vi "niDTS WLAN UTIL chains to chains array.vi"(10 "Chains":T1) -> (2 "Chains Array":bool[](array[boolean])=[TRUE, FALSE, FALSE, FALSE])   [LabVIEW 2014, in "niDTS WLAN.lvlib"]
uses:
  niDTS WLAN.lvlib
  Includes/niDTS WLAN INC Chains.ctl
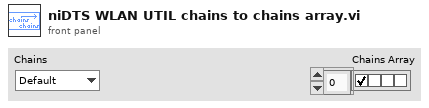
[diagram p1: front panel]
types:
  T1 = typedef "niDTS WLAN.lvlib/niDTS WLAN INC Chains.ctl" = enum16{"Default", "Chain 0", "Chain 1", "Chain 2", "Chain 3", "Chain 0 and 1", "Chain 2 and 3", "Chain 1,2 and 3", "Chains 1 - 4"}
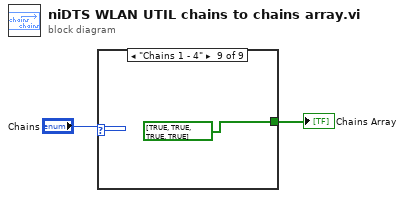
[diagram p0: block diagram]
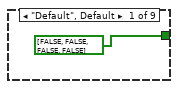
[diagram p2: hidden frame]
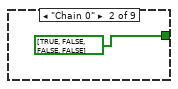
[diagram p3: hidden frame]
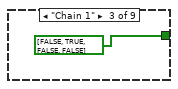
[diagram p4: hidden frame]
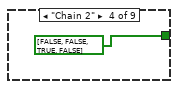
[diagram p5: hidden frame]
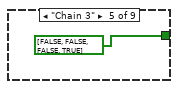
[diagram p6: hidden frame]
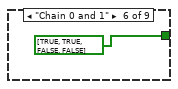
[diagram p7: hidden frame]
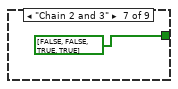
[diagram p8: hidden frame]
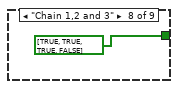
[diagram p9: hidden frame]
diagram:
  n1 = case shown="\"Chains 1 - 4\"" "Chains" {
    tunnel: [bool[] [FALSE, FALSE, FALSE, FALSE] bool[] [TRUE, FALSE, FALSE, FALSE] bool[] [FALSE, TRUE, FALSE, FALSE] bool[] [FALSE, FALSE, TRUE, FALSE] bool[] [FALSE, FALSE, FALSE, TRUE] bool[] [TRUE, TRUE, FALSE, FALSE] bool[] [FALSE, FALSE, TRUE, TRUE] bool[] [TRUE, TRUE, TRUE, FALSE] bool[] [TRUE, TRUE, TRUE, TRUE]] -> w1
    frame "Default", Default {
    }
    frame "Chain 0" {
    }
    frame "Chain 1" {
    }
    frame "Chain 2" {
    }
    frame "Chain 3" {
    }
    frame "Chain 0 and 1" {
    }
    frame "Chain 2 and 3" {
    }
    frame "Chain 1,2 and 3" {
    }
    frame "Chains 1 - 4" {
    }
  }
  "Chains Array" <- w1
